vi "GetVersionSerializableData_StaticCommunity.vi"(10 "Version":u16, 11 "BlueSerializable in":refnum<class "BlueSerializable.lvclass">) -> (0 "error out":errorcluster, 1 "Found?":bool, 2 "SerializableData":variant, 3 "BlueSerializable out":refnum<class "BlueSerializable.lvclass">)   [LabVIEW 2020, in "BlueSerialization.lvlib" / "BlueSerializable.lvclass"]
uses:
  BlueSerializable.lvclass
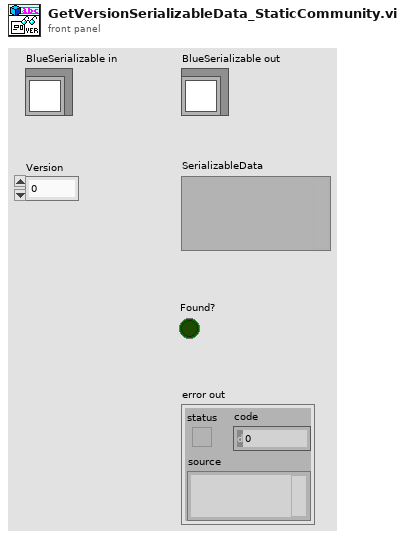
[diagram p1: front panel]
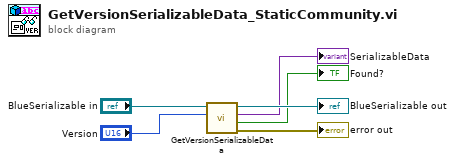
[diagram p0: block diagram]
diagram:
  n1 = call-dynamic "GetVersionSerializableData.vi"("Version"="Version", "BlueSerializable in"="BlueSerializable in") -> ("error out"=→"error out":errorcluster, "Found?"=→"Found?":bool, "SerializableData"=→"SerializableData":variant, "BlueSerializable out"=→"BlueSerializable out":refnum<class "BlueSerializable.lvclass">)  [unwired: 6 in]
